vi "Module Reset.vi"(8 "error in (no error)":errorcluster, 10 "ModuleName":string="unnamed", 11 "Mod Admin in":refnum<class "ModuleAdmin.lvclass">) -> (0 "error out":errorcluster, 3 "Mod Admin out":refnum<class "ModuleAdmin.lvclass">)   [LabVIEW 2014, in "ModuleAdmin.lvlib" / "ModuleAdmin.lvclass"]
uses:
  ModuleAdmin.lvclass
  ModuleAdmin.lvclass/ModuleAdmin.ctl
  Accessors/Write ShowPanel_.vi
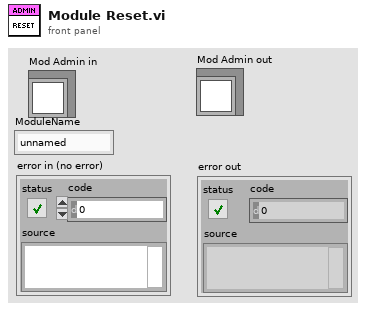
[diagram p1: front panel]
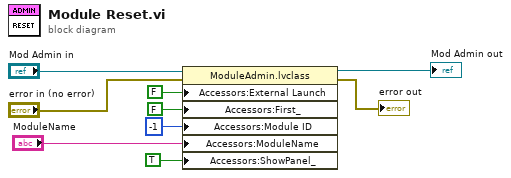
[diagram p0: block diagram]
diagram:
  n1 = property class="ModuleAdmin.lvclass"(reference="Mod Admin in", error in="error in (no error)", "Accessors:External Launch"=FALSE ("External Launch"), "Accessors:First_"=FALSE ("First_"), "Accessors:Module ID"=-1 ("Module ID"), "Accessors:ModuleName"="ModuleName", "Accessors:ShowPanel_"=TRUE) -> (reference out=→"Mod Admin out":refnum<class "ModuleAdmin.lvclass">, error out=→"error out":errorcluster)
